vi "Arrange VIWin - Order FP Conn Pane Controls.vi"(0 "controls in":refnum<vi>[](array[refnum]), 5 "terminal bounds":T2[](array[typedef])) -> (4 "sorted controls":refnum<vi>[](array[refnum]), 6 "sorted terminal boundaries":T2[](array[typedef]), 8 "sorted array of control info":T1[](array[typedef]))   [LabVIEW 2015, in "Arrange VI Window.lvlib"]
uses:
  Arrange VI Window.lvlib
  <vilib>/Utility/miscctls.llb/LVRectTypeDef.ctl
  Arrange VIWin - FP Control Info.ctl
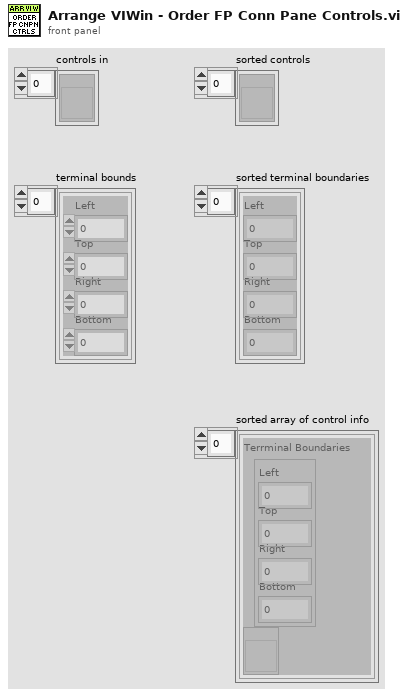
[diagram p1: front panel]
types:
  T1 = typedef "Arrange VI Window.lvlib/Arrange VIWin - FP Control Info.ctl" = cluster{"Terrminal Boundaries":T2, "Control Reference":refnum<vi>}
  T2 = typedef "LVRectTypeDef.ctl" = cluster{"Left":i16, "Top":i16, "Right":i16, "Bottom":i16}
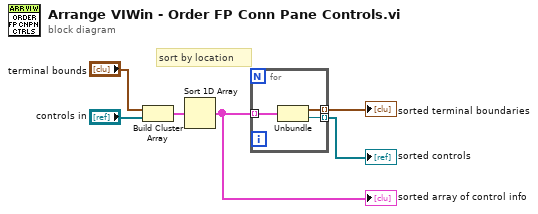
[diagram p0: block diagram]
diagram:
  # "sort by location"
  n1 = Build Cluster Array("terminal bounds", "controls in") -> (w4:cluster{"Rectangle":T2, refnum<vi>}[])
  n2 = Sort 1D Array(array=w4) -> (sorted array=w3:cluster{"Rectangle":T2, refnum<vi>}[])
  "sorted array of control info" <- w3
  n3 = for {
    tunnel: w3 -> [w9] mode=indexing
    tunnel: [w8] -> w6 mode=indexing
    tunnel: [w7] -> w5 mode=indexing
    n4 = Unbundle(w9) -> ("Rectangle"=w7:T2, w8:refnum<vi>)
  }
  "sorted terminal boundaries" <- w5
  "sorted controls" <- w6
